vi "SetSystemTime.vi"(8 "error in (no error)":errorcluster, 11 "Time In":timestamp) -> (0 "error out":errorcluster)   [LabVIEW 2020]
uses:
  kernel32.dll
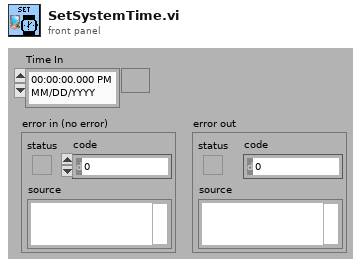
[diagram p1: front panel]
types:
  T1 = cluster{"Year":i16, "Month":i16, "Day of Week":i16, "Day of Month":i16, "Hour":i16, "Minute":i16, "Second":i16, "Millisecond":i16}
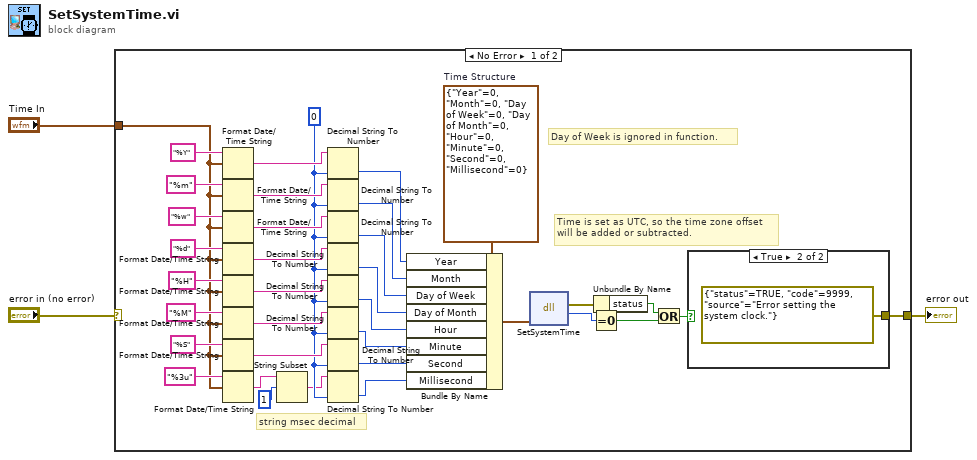
[diagram p0: block diagram]
diagram:
  n1 = case shown="No Error" "error in (no error)" {
    selector: "error in (no error)" -> [_ w41]
    tunnel: [w8 w41] -> w3
    tunnel: "Time In" -> [w29 _]
    frame No Error {
      w20 = i16 0 ("default (0 I32)")
      w39 = T1 {"Year"=0, "Month"=0, "Day of Week"=0, "Day of Month"=0, "Hour"=0, "Minute"=0, "Second"=0, "Millisecond"=0}  # Time Structure
      # "Time is set as UTC, so the time zone offset\nwill be added or subtracted."
      # "string msec decimal"
      # "Day of Week is ignored in function."
      n2 = Format Date/Time String(time format string (%c)="%Y", seconds (now)=w29) -> (date/time string=w28:string)  [unwired: 1 in]
      n3 = Format Date/Time String(time format string (%c)="%m", seconds (now)=w29) -> (date/time string=w26:string)  [unwired: 1 in]
      n4 = Format Date/Time String(time format string (%c)="%w", seconds (now)=w29) -> (date/time string=w25:string)  [unwired: 1 in]
      n5 = Format Date/Time String(time format string (%c)="%d", seconds (now)=w29) -> (date/time string=w24:string)  [unwired: 1 in]
      n6 = Format Date/Time String(time format string (%c)="%H", seconds (now)=w29) -> (date/time string=w23:string)  [unwired: 1 in]
      n7 = Format Date/Time String(time format string (%c)="%M", seconds (now)=w29) -> (date/time string=w22:string)  [unwired: 1 in]
      n8 = Format Date/Time String(time format string (%c)="%S", seconds (now)=w29) -> (date/time string=w21:string)  [unwired: 1 in]
      n9 = Format Date/Time String(time format string (%c)="%3u", seconds (now)=w29) -> (date/time string=w12:string)  [unwired: 1 in]
      n10 = String Subset(string=w12, offset (0)=1) -> (substring=w10:string)  [unwired: 1 in]
      n11 = Decimal String To Number(string=w28, default (0L)=w20) -> (number=w27:i16)  [unwired: 1 in, 1 out]
      n12 = Decimal String To Number(string=w26, default (0L)=w20) -> (number=w19:i16)  [unwired: 1 in, 1 out]
      n13 = Decimal String To Number(string=w25, default (0L)=w20) -> (number=w18:i16)  [unwired: 1 in, 1 out]
      n14 = Decimal String To Number(string=w24, default (0L)=w20) -> (number=w17:i16)  [unwired: 1 in, 1 out]
      n15 = Decimal String To Number(string=w23, default (0L)=w20) -> (number=w16:i16)  [unwired: 1 in, 1 out]
      n16 = Decimal String To Number(string=w22, default (0L)=w20) -> (number=w15:i16)  [unwired: 1 in, 1 out]
      n17 = Decimal String To Number(string=w21, default (0L)=w20) -> (number=w14:i16)  [unwired: 1 in, 1 out]
      n18 = Decimal String To Number(string=w10, default (0L)=w20) -> (number=w13:i16)  [unwired: 1 in, 1 out]
      n19 = Bundle By Name(cluster=w39, "Year"=w27, "Month"=w19, "Day of Week"=w18, "Day of Month"=w17, "Hour"=w16, "Minute"=w15, "Second"=w14, "Millisecond"=w13) -> (w38:T1)
      n20 = dll-call lib="kernel32.dll" fn="SetSystemTime"("TimeStructureIn"=w38) -> (error out=w7:errorcluster, "return type"=w9:i8)  [unwired: 4 in, 1 out]
      n21 = Equal To 0?(x=w9) -> (x = 0?=w4:bool)
      n22 = Unbundle By Name(w7) -> ("status"=w5:bool)
      n23 = Or(x=w5, y=w4) -> (x .or. y?=w6:bool)
      n24 = case shown="True" w6 {
        tunnel: [_ errorcluster {"status"=TRUE, "code"=9999, "source"="Error setting the system clock."} ("error out 2")] -> w8
        frame False {
        }
        frame True {
        }
      }
    }
    frame Error {
    }
  }
  "error out" <- w3
